vi "LOOP.vi"() -> ()   [LabVIEW 2017]
panel:
  out "Boolean":bool
  out "Slide":u8(slide) scale=0.0..100.0
  out "Meter":dbl(knob) scale=0.0..100.0
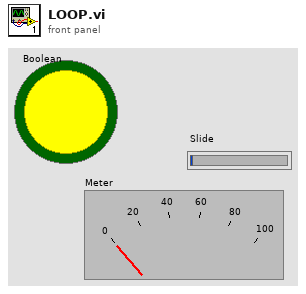
[diagram p1: front panel]
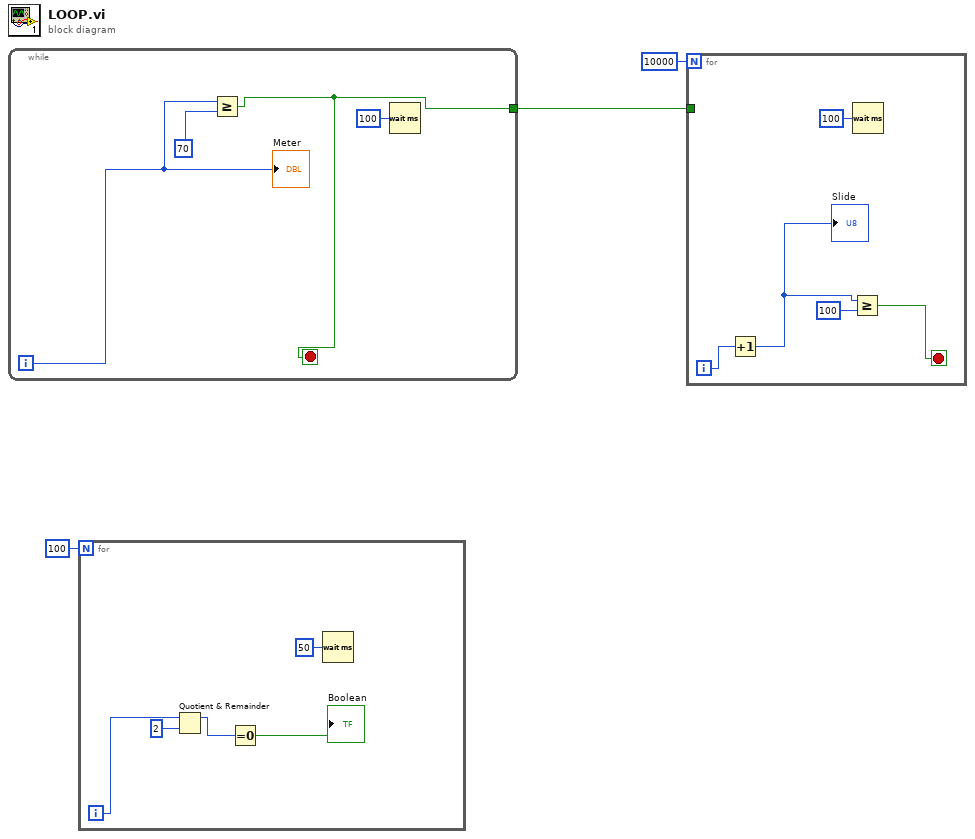
[diagram p0: block diagram]
diagram:
  n1 = while {
    tunnel: [w4] -> w2
    i -> [w5]
    stop <- w4 stop-if-true
    n2 = Greater Or Equal?(x=w5, y=70) -> (x >= y?=w4:bool)
    n3 = Wait (ms)(milliseconds to wait=u32 100) -> ()  [unwired: 1 out]
    "Meter" <- w5
  }
  n4 = for {
    N: 100 -> [_]
    i -> [w11]
    n5 = Quotient & Remainder(x=w11, y=2) -> (x-y*floor(x/y)=w9:i32)  [unwired: 1 out]
    n6 = Equal To 0?(x=w9) -> (x = 0?=→"Boolean":bool)
    n7 = Wait (ms)(milliseconds to wait=u32 50) -> ()  [unwired: 1 out]
  }
  n8 = for {
    N: 10000 -> [_]
    tunnel: w2 -> [_]
    i -> [w17]
    stop <- w14 stop-if-true
    n9 = Increment(x=w17) -> (x+1=w16:i32)
    "Slide" <- w16
    n10 = Greater Or Equal?(x=w16, y=100) -> (x >= y?=w14:bool)
    n11 = Wait (ms)(milliseconds to wait=u32 100) -> ()  [unwired: 1 out]
  }
